vi "Destroy User Events.vi"(8 "error in (no error)":errorcluster, 11 "Generador de Señales in":refnum<class "Generador de Señales.lvclass">) -> (0 "error out":errorcluster, 3 "Generador de Señales out":refnum<class "Generador de Señales.lvclass">)   [LabVIEW 2020, in "Generador de Señales.lvlib" / "Generador de Señales.lvclass"]
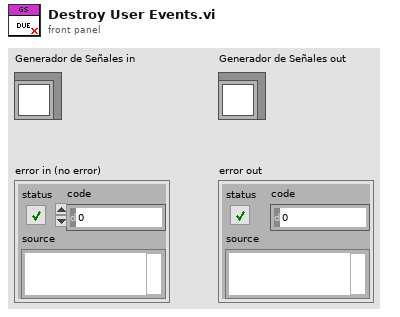
[diagram p1: front panel]
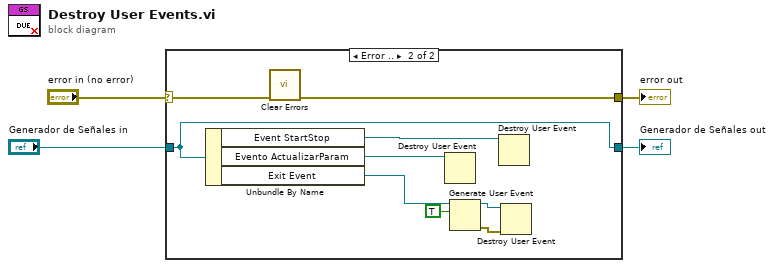
[diagram p0: block diagram]
diagram:
  n1 = case shown="Error .." "error in (no error)" {
    selector: "error in (no error)" -> [w5 w11]
    tunnel: [w5 w12] -> w1
    tunnel: [w6 w15] -> w2
    tunnel: "Generador de Señales in" -> [w6 w15]
    frame No Error {
    }
    frame Error {
      n2 = Unbundle By Name(w15) -> ("Event StartStop"=w13:refnum<user-event>, "Evento ActualizarParam"=w14:refnum<user-event>, "Exit Event"=w10:refnum<user-event>)
      n3 = call <vilib>:"Clear Errors.vi"("error in (no error)"=w11) -> ("error out"=w12:errorcluster)  [unwired: 5 in, 1 out]
      n4 = Destroy User Event(user event=w14) -> ()  [unwired: 1 in, 1 out]
      n5 = Generate User Event(user event=w10, event data cluster=TRUE ("event data")) -> (user event out=w8:refnum<user-event>, error out=w7:errorcluster)  [unwired: 2 in]
      n6 = Destroy User Event(user event=w13) -> ()  [unwired: 1 in, 1 out]
      n7 = Destroy User Event(user event=w8, error in=w7) -> ()  [unwired: 1 out]
    }
  }
  "Generador de Señales out" <- w2
  "error out" <- w1
